vi "LPC basic command line.vi"() -> ()   [LabVIEW 2009, in "BEOC LPC.lvlib"]
uses:
  <vilib>/Instr/_visa.llb/GPIB Status Boolean Array.ctl
  BEOC LPC.lvlib
panel:
  in  "bytes to request":i32=1024
  out "response":string
  out "ibsta 2":T1
  in  "command":string
  out "ibsta":T1
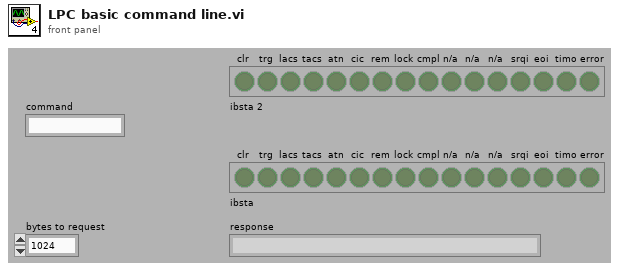
[diagram p1: front panel]
types:
  T1 = typedef "GPIB Status Boolean Array.ctl" = bool[]
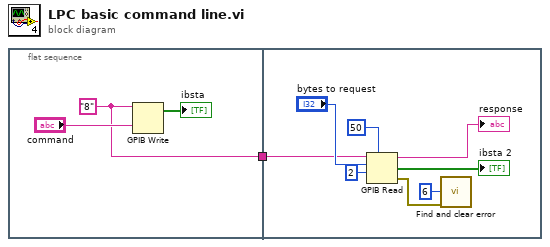
[diagram p0: block diagram]
diagram:
  n1 = flat-sequence {
    tunnel: [w2] -> w1
    tunnel: w1 -> [w9]
    frame #0 {
      w2 = "8" ("address string")
      n2 = GPIB Write(0:w2, 1:"command") -> (5:→"ibsta":bool[])  [unwired: 1 in, 3 out]
    }
    frame #1 {
      n3 = GPIB Read(0:w9, 1:"bytes to request", 2:i16 2 ("mode (0)"), 4:50 ("timeout ms (488.2 global)")) -> (5:→"response":string, 6:→"ibsta 2":bool[], 7:w7:errorcluster)  [unwired: 1 in]
      n4 = call "Find and clear error.vi"("error in (no error)"=w7, "error code"=6) -> ()  [unwired: 10 out]
    }
  }
